vi "HardwareConfiguration.vi"() -> (3 "configured?":bool)   [LabVIEW 2018]
uses:
  InstrControl/InstrumentSetup.vi
  globals/QC_RunInformation.vi
  InstrControl/InstrControl.lvclass
panel:
  in  "Preferences Button":bool
  in  "Defaults Multimeter":bool
  in  "Multimeter":enum32{"Keithley 2000"}(tab)
  in  "Range Value\n(0.1 - 100)":dbl=100.0 format="%#.2g"
  in  "Range":u16(ring) items=["Auto", "Manual"]
  in  "Function":u16(ring)=3 items=["AC Current", "DC Current", "AC Voltage", "DC Voltage", "2W-Resistance", "4W-Resistance", "Period", "Frequency", "Temperature", "Diode", "Continuity"]
  in  "GPIB Address KE2000":string
  in  "Defaults LCR":bool
  in  "LCRs":enum32{"WayneKerr 6440B", "WayneKerr 6425"}(tab)
  in  "AC frequency [Hz]":i32=1000 format="%#.3p"
  in  "RC Configuration":u16(ring) items=["serial", "parallel"]
  in  "AC amplitude [V]":sgl=0.1
  in  "GPIB Address WK6440B":string
  in  "GPIB Address WK6425":string
  in  "AC amplitude [V] WK6425":sgl=0.1 caption="AC amplitude [V]"
  in  "RC Configuration WK6425":u16(ring) caption="RC Configuration" items=["serial", "parallel"]
  in  "AC frequency [Hz] WK6425":i32=1000 caption="AC frequency [Hz]" format="%#.3p"
  in  "VISA address":refnum<visa-resource-name>="COM24" caption="Arduino address"
  out "Programm uploaded?":string="Make sure programme is uploaded to Arduino Uno ->"
  in  "Blank Button":bool
  in  "Supplies":T1(tab)
  in  "Current Limit [µA]":sgl=100.0
  in  "GPIB Address KE2410":string
  in  "GPIB Address KE487":string
  in  "Compliance":u16(ring) items=["20µA", "2mA"]
  in  "Range:":u16(ring) items=["Autorange", "2nA", "20nA", "200nA", "2 microAmp", "20 microAmp", "200 microAmp", "2 milliAmp"]
  in  "Current Limit":u16(ring)=1 items=["OFF", "ON"]
  in  "GPIB Address KE6517":string
  in  "current compliance \nlevel [mA]":dbl=0.0001 format="%.4f"
  in  "compliance/measurement\nrange (auto:0)":u16(ring)=6 items=["auto / auto", "1 nA / 1.1 V", "10 nA / 11 V", "100 nA / 110 V", "0.001 mA / 110 V", "0.01 mA / 110 V", "0.1 mA / 110 V", "1 mA / 110 V", "10 mA / 110 V", "100 mA / 110 V"]
  in  "GPIB Address KE236":string
  in  "Defaults Supply":bool
  in  "OK Button":bool
  # "Hardware Configuration"
  # "Multimeter Configuration"
  # "Supply Configuration"
  # "Arduino Configuration"
  # "LCR Configuration"
  # "(Only for initialisation)"
  # "(Only for initialisation)"
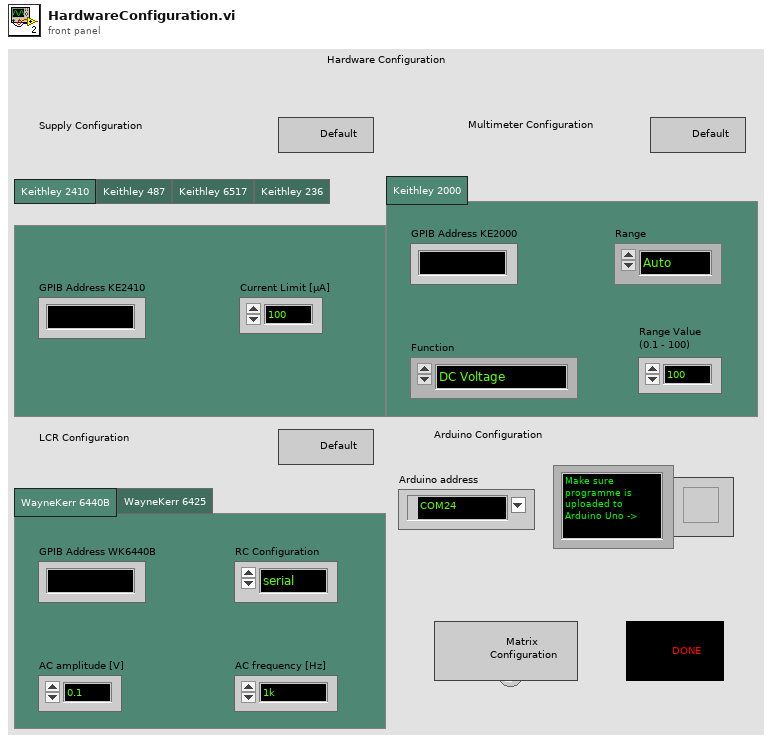
[diagram p1: front panel]
types:
  T1 = enum32{"Keithley 2410", "Keithley 487", "Keithley 6517", "Keithley 236"}
  T2 = cluster{"VISA address":refnum<visa-resource-name>, "T sensor":enum16{"SHT", "DS"}, "Arduino":refnum<class "ArduinoControl.lvclass">}
  T3 = cluster{"KE 2410":cluster{"Instrument name":string, "GPIB address":string, "Instrument type":u16}, "KE 6517":cluster{"Instrument name":string, "GPIB address":string, "Instrument type":u16}, "KE 487":cluster{"Instrument name":string, "GPIB address":string, "Instrument type":u16}, "KE 487_2":cluster{"Instrument name":string, "GPIB address":string, "Instrument type":u16}, "KE 236":cluster{"Instrument name":string, "GPIB address":string, "Instrument type":u16}, "WK 6440B":cluster{"Instrument name":string, "GPIB address":string, "Instrument type":u16}, "WK 6425":cluster{"Instrument name":string, "GPIB address":string, "Instrument type":u16}, "Pickering Matrix":cluster{"Instrument name":string, "GPIB address":string, "Instrument type":u16}, "KE 2000":cluster{"Instrument name":string, "GPIB address":string, "Instrument type":u16}, "KE 2657A":cluster{"Instrument name":string, "GPIB address":string, "Instrument type":u16}}
  T4 = cluster{"Sensor Serial No.:":string, "Wafer Serial No.:":string, "Batch:":string, "Manufacturer:":string, "Device Category:":string, "Database Serial No.:":string, "Initiated:":string, "Test":string, "Instruments used:":string, "Probeplan used:":string, "End of Run comment:":string, "User:":string}
  T5 = cluster{"RC Configuration":u16, "AC amplitude [V]":dbl, "AC frequency [Hz]":i32, "WK6440B":refnum<class "WK6440B.lvclass">}
  T6 = cluster{"RC Configuration":u16, "AC amplitude [V]":dbl, "AC frequency [Hz]":i32, "WK6425":refnum<class "WK6425.lvclass">}
  T7 = cluster{"Range":u16, "Range Value":dbl, "Function":u16, "KE2000":refnum<class "KE2000.lvclass">}
  T8 = cluster{"Current Limit":sgl, "KE2410":refnum<class "KE2410.lvclass">}
  T9 = cluster{"Compliance":u16, "Range:":u16, "KE487":refnum<class "KE487.lvclass">}
  T10 = cluster{"Current Limit":u16, "KE6517":refnum<class "KE6517.lvclass">}
  T11 = cluster{"current \ncompliance level":dbl, "compliance/\nmeasurement range (auto:0)":u16, "KE236":refnum<class "KE236.lvclass">}
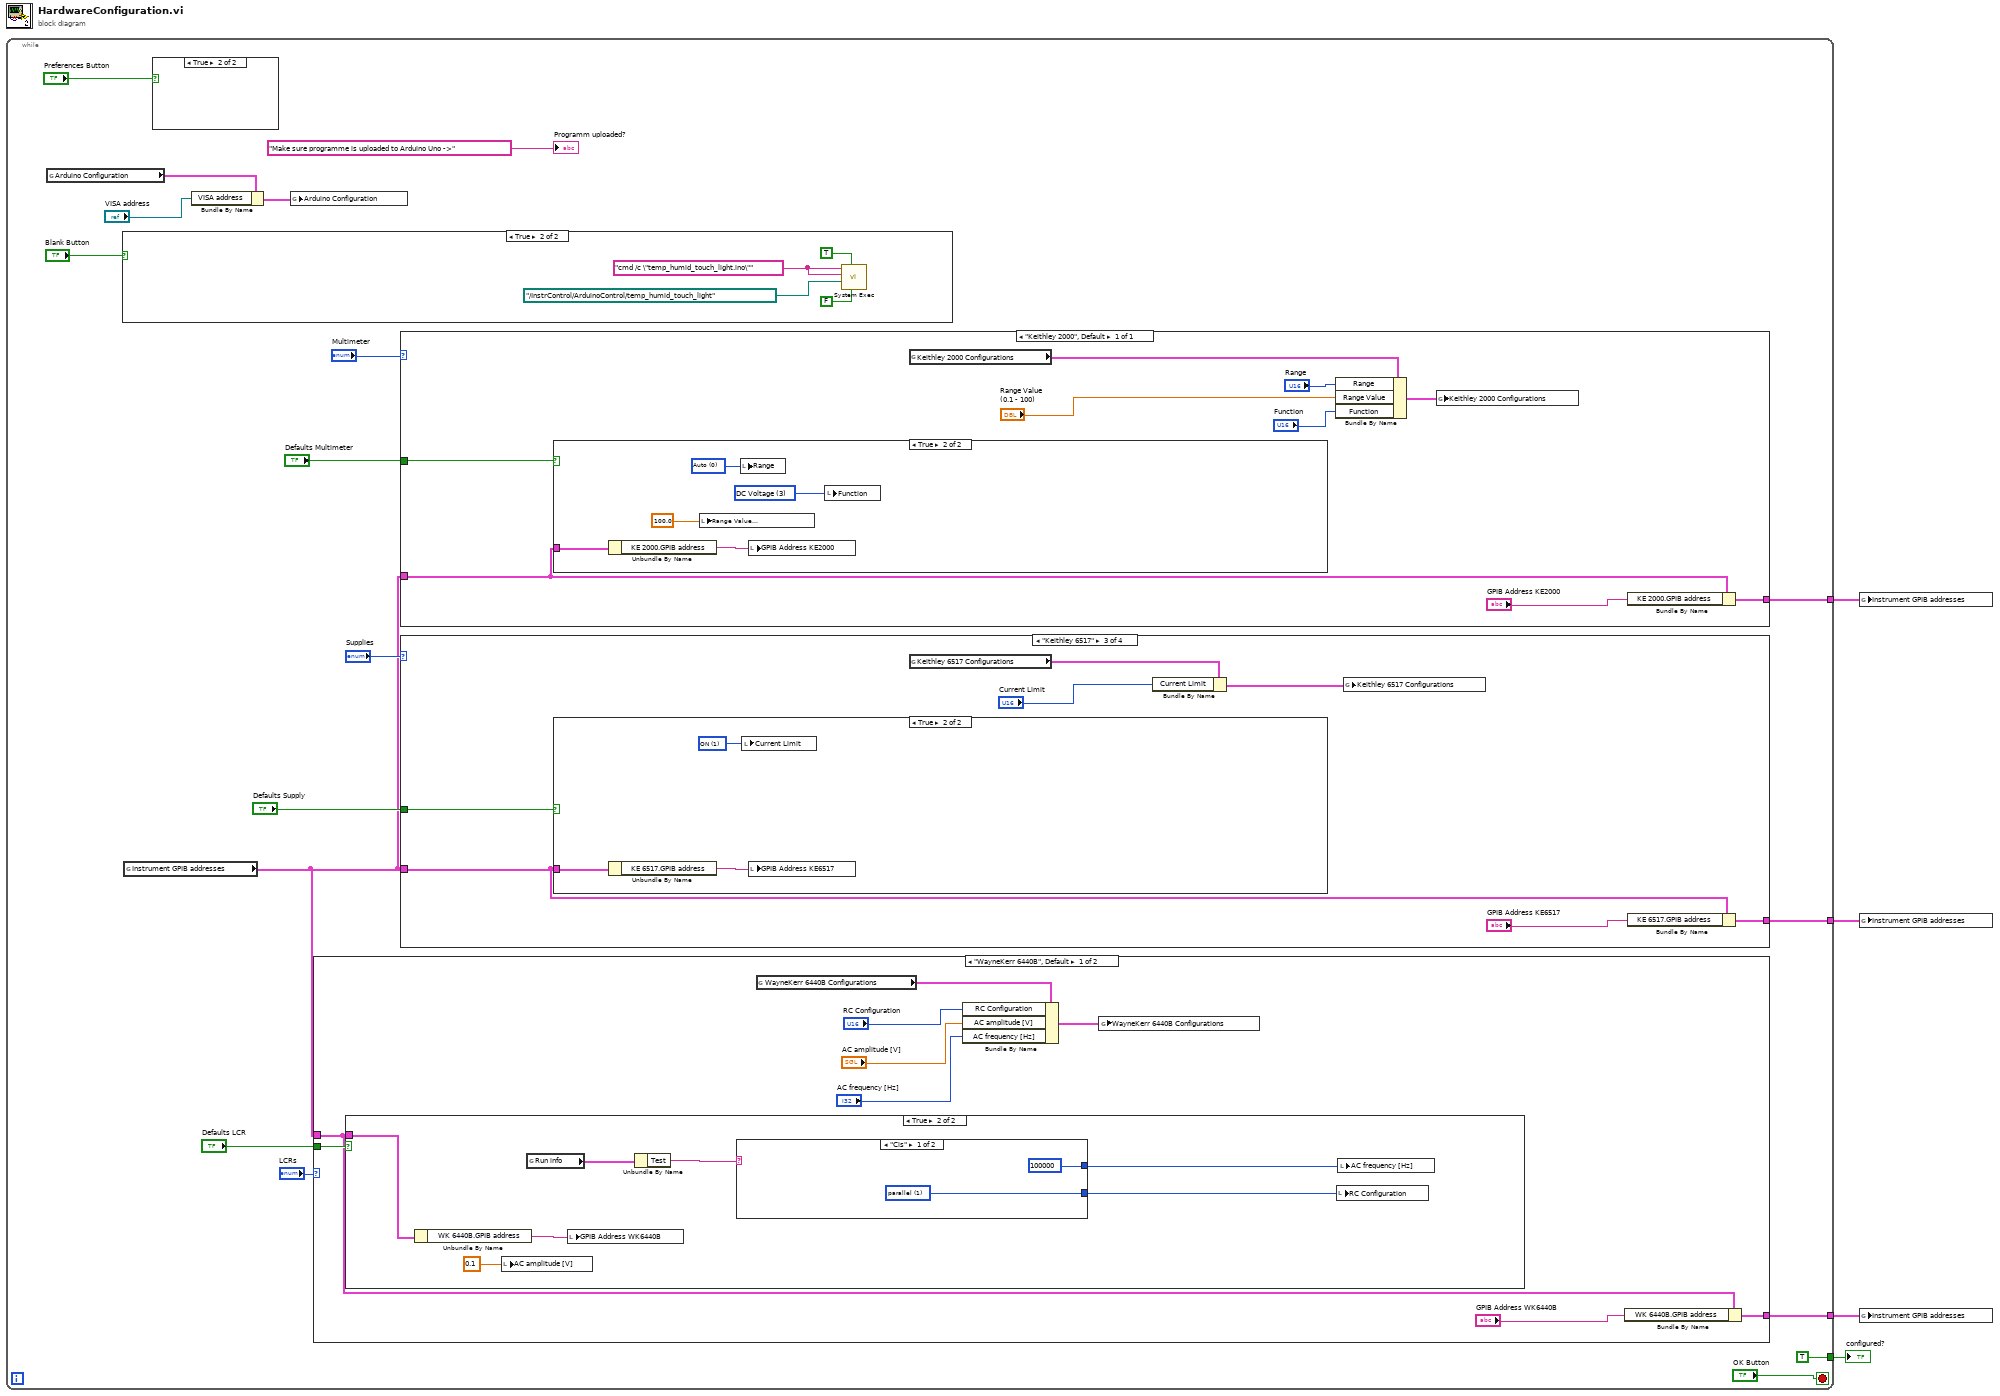
[diagram p0: block diagram]
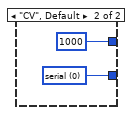
[diagram p6: hidden frame]
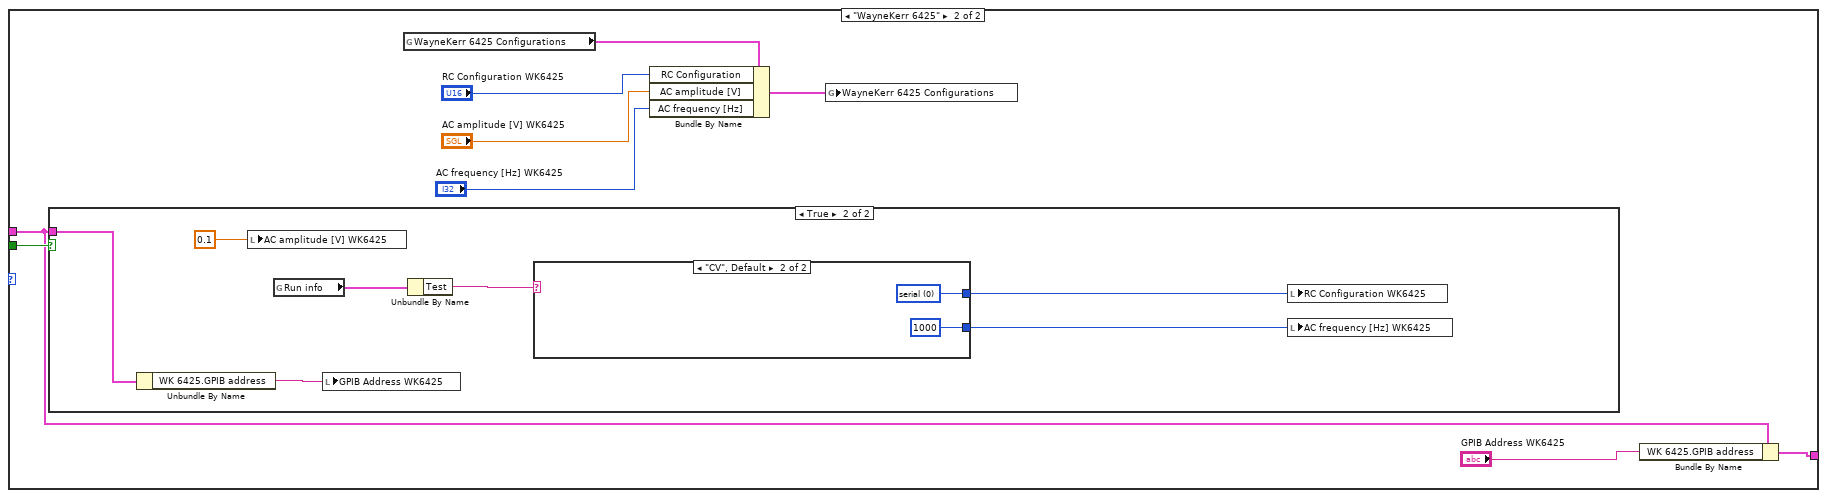
[diagram p7: hidden frame]
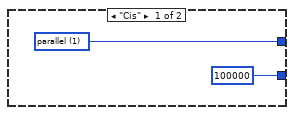
[diagram p9: hidden frame]
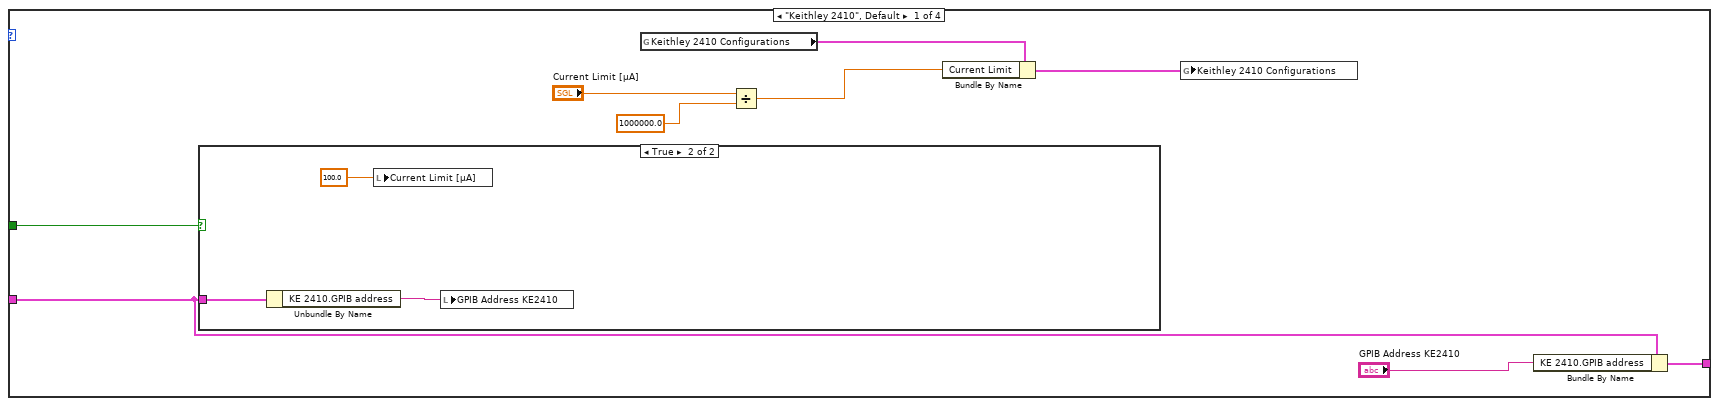
[diagram p10: hidden frame]
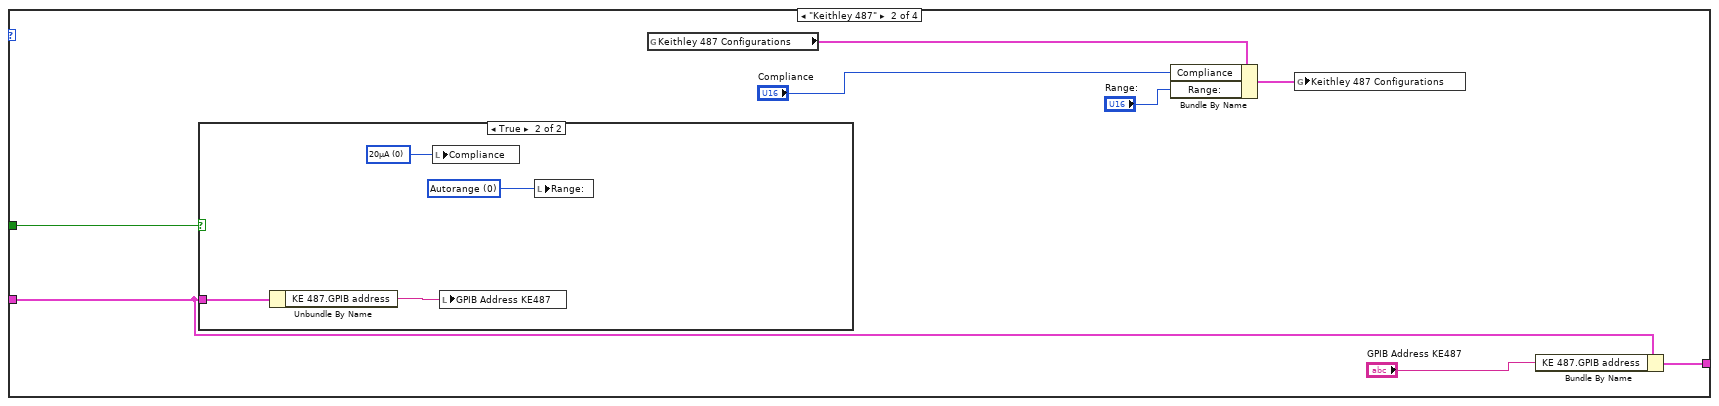
[diagram p12: hidden frame]
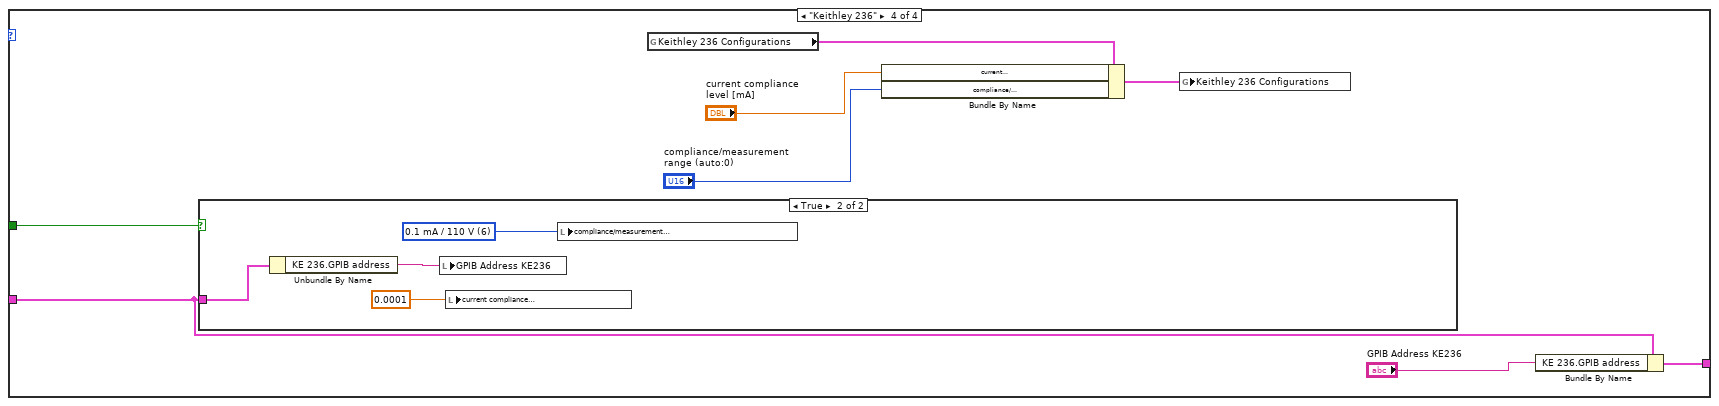
[diagram p15: hidden frame]
diagram:
  n1 = while {
    tunnel: [w9] -> w4
    tunnel: [w8] -> w3
    tunnel: [w7] -> w2
    tunnel: [TRUE] -> w1
    stop <- "OK Button" stop-if-true
    n2 = global read "InstrumentSetup.vi" "Arduino Configuration"() -> (w12:T2)
    n3 = case shown="True" "Blank Button" {
      frame False {
      }
      frame True {
        w24 = "cmd /c \"temp_humid_touch_light.ino\""
        n4 = call <vilib>:"System Exec.vi"("run minimized? (F)"=FALSE, "wait until completion? (T)"=TRUE, "working directory"=path "../InstrControl/ArduinoControl/temp_humid_touch_light", "standard input"=w24, "command line"=w24) -> ()  [unwired: 3 in, 4 out]
      }
    }
    n5 = global read "InstrumentSetup.vi" "Instrument GPIB addresses"() -> (w17:T3)
    n6 = case shown="True" "Preferences Button" {
      frame False {
      }
      frame True {
      }
    }
    n7 = Bundle By Name(cluster=w12, "VISA address"="VISA address") -> (w11:T2)
    n8 = global write "InstrumentSetup.vi" "Arduino Configuration"(w11) -> ()
    n9 = case shown="\"WayneKerr 6440B\", Default" "LCRs" {
      tunnel: "Defaults LCR" -> [w47 w67]
      tunnel: w17 -> [w46 w66]
      tunnel: [w45 w65] -> w9
      frame "WayneKerr 6440B", Default {
        n10 = case shown="True" w47 {
          tunnel: w46 -> [_ w56]
          frame False {
          }
          frame True {
            n11 = Unbundle By Name(w56) -> ("WK 6440B.GPIB address"=w50:string)
            n12 = local write "AC amplitude [V]"(0.1) -> ()
            n13 = global read "QC_RunInformation.vi" "Run info"() -> (w52:T4)
            n14 = local write "GPIB Address WK6440B"(w50) -> ()
            n15 = Unbundle By Name(w52) -> ("Test"=w51:string)
            n16 = case shown="\"Cis\"" w51 {
              tunnel: [w58 w60] -> w54
              tunnel: [100000 1000] -> w53
              frame "Cis" {
                w58 = u16 1 items=["serial", "parallel"] ("RC Configuration")
              }
              frame "CV", Default {
                w60 = u16 0 items=["serial", "parallel"] ("RC Configuration")
              }
            }
            n17 = local write "RC Configuration"(w54) -> ()
            n18 = local write "AC frequency [Hz]"(w53) -> ()
          }
        }
        n19 = global read "InstrumentSetup.vi" "WayneKerr 6440B Configurations"() -> (w49:T5)
        n20 = Bundle By Name(cluster=w49, "RC Configuration"="RC Configuration", "AC amplitude [V]"="AC amplitude [V]", "AC frequency [Hz]"="AC frequency [Hz]") -> (w48:T5)
        n21 = global write "InstrumentSetup.vi" "WayneKerr 6440B Configurations"(w48) -> ()
        n22 = Bundle By Name(cluster=w46, "WK 6440B.GPIB address"="GPIB Address WK6440B") -> (w45:T3)
      }
      frame "WayneKerr 6425" {
        n23 = case shown="True" w67 {
          tunnel: w66 -> [_ w76]
          frame False {
          }
          frame True {
            n24 = Unbundle By Name(w76) -> ("WK 6425.GPIB address"=w70:string)
            n25 = local write "AC amplitude [V] WK6425"(0.1) -> ()
            n26 = global read "QC_RunInformation.vi" "Run info"() -> (w72:T4)
            n27 = local write "GPIB Address WK6425"(w70) -> ()
            n28 = Unbundle By Name(w72) -> ("Test"=w71:string)
            n29 = case shown="\"CV\", Default" w71 {
              tunnel: [w78 w80] -> w74
              tunnel: [100000 1000] -> w73
              frame "Cis" {
                w78 = u16 1 items=["serial", "parallel"] ("RC Configuration")
              }
              frame "CV", Default {
                w80 = u16 0 items=["serial", "parallel"] ("RC Configuration")
              }
            }
            n30 = local write "RC Configuration WK6425"(w74) -> ()
            n31 = local write "AC frequency [Hz] WK6425"(w73) -> ()
          }
        }
        n32 = global read "InstrumentSetup.vi" "WayneKerr 6425 Configurations"() -> (w69:T6)
        n33 = Bundle By Name(cluster=w69, "RC Configuration"="RC Configuration WK6425", "AC amplitude [V]"="AC amplitude [V] WK6425", "AC frequency [Hz]"="AC frequency [Hz] WK6425") -> (w68:T6)
        n34 = global write "InstrumentSetup.vi" "WayneKerr 6425 Configurations"(w68) -> ()
        n35 = Bundle By Name(cluster=w66, "WK 6425.GPIB address"="GPIB Address WK6425") -> (w65:T3)
      }
    }
    n36 = case shown="\"Keithley 2000\", Default" "Multimeter" {
      tunnel: "Defaults Multimeter" -> [w35]
      tunnel: w17 -> [w32]
      tunnel: [w31] -> w7
      frame "Keithley 2000", Default {
        n37 = case shown="True" w35 {
          tunnel: w32 -> [_ w40]
          frame False {
          }
          frame True {
            w38 = u16 0 items=["Auto", "Manual"] ("Range")
            w39 = u16 3 items=["AC Current", "DC Current", "AC Voltage", "DC Voltage", "2W-Resistance", "4W-Resistance", "Period", "Frequency", "Temperature", "Diode", "Continuity"] ("Function")
            n38 = Unbundle By Name(w40) -> ("KE 2000.GPIB address"=w36:string)
            n39 = local write "Range Value\n(0.1 - 100)"(100.0 ("Range Value\n(0.1 - 100)")) -> ()
            n40 = local write "Range"(w38) -> ()
            n41 = local write "GPIB Address KE2000"(w36) -> ()
            n42 = local write "Function"(w39) -> ()
          }
        }
        n43 = global read "InstrumentSetup.vi" "Keithley 2000 Configurations"() -> (w34:T7)
        n44 = Bundle By Name(cluster=w34, "Range"="Range", "Range Value"="Range Value\n(0.1 - 100)", "Function"="Function") -> (w33:T7)
        n45 = global write "InstrumentSetup.vi" "Keithley 2000 Configurations"(w33) -> ()
        n46 = Bundle By Name(cluster=w32, "KE 2000.GPIB address"="GPIB Address KE2000") -> (w31:T3)
      }
    }
    n47 = case shown="\"Keithley 6517\"" "Supplies" {
      tunnel: "Defaults Supply" -> [w89 w100 w111 w122]
      tunnel: w17 -> [w83 w97 w108 w118]
      tunnel: [w84 w96 w107 w119] -> w8
      frame "Keithley 2410", Default {
        n48 = case shown="True" w89 {
          tunnel: w83 -> [_ w92]
          frame False {
          }
          frame True {
            n49 = Unbundle By Name(w92) -> ("KE 2410.GPIB address"=w90:string)
            n50 = local write "Current Limit [µA]"(100.0) -> ()
            n51 = local write "GPIB Address KE2410"(w90) -> ()
          }
        }
        n52 = global read "InstrumentSetup.vi" "Keithley 2410 Configurations"() -> (w88:T8)
        n53 = Divide(x="Current Limit [µA]", y=1000000.0) -> (x/y=w85:dbl)
        n54 = Bundle By Name(cluster=w88, "Current Limit"=w85) -> (w87:T8)
        n55 = global write "InstrumentSetup.vi" "Keithley 2410 Configurations"(w87) -> ()
        n56 = Bundle By Name(cluster=w83, "KE 2410.GPIB address"="GPIB Address KE2410") -> (w84:T3)
      }
      frame "Keithley 487" {
        n57 = case shown="True" w100 {
          tunnel: w97 -> [_ w104]
          frame False {
          }
          frame True {
            w102 = u16 0 items=["Autorange", "2nA", "20nA", "200nA", "2 microAmp", "20 microAmp", "200 microAmp", "2 milliAmp"] ("Range:")
            w103 = u16 0 items=["20µA", "2mA"] ("Compliance")
            n58 = Unbundle By Name(w104) -> ("KE 487.GPIB address"=w101:string)
            n59 = local write "Compliance"(w103) -> ()
            n60 = local write "GPIB Address KE487"(w101) -> ()
            n61 = local write "Range:"(w102) -> ()
          }
        }
        n62 = global read "InstrumentSetup.vi" "Keithley 487 Configurations"() -> (w99:T9)
        n63 = Bundle By Name(cluster=w99, "Compliance"="Compliance", "Range:"="Range:") -> (w98:T9)
        n64 = global write "InstrumentSetup.vi" "Keithley 487 Configurations"(w98) -> ()
        n65 = Bundle By Name(cluster=w97, "KE 487.GPIB address"="GPIB Address KE487") -> (w96:T3)
      }
      frame "Keithley 6517" {
        n66 = case shown="True" w111 {
          tunnel: w108 -> [_ w114]
          frame False {
          }
          frame True {
            w113 = u16 1 items=["OFF", "ON"] ("Current Limit")
            n67 = Unbundle By Name(w114) -> ("KE 6517.GPIB address"=w112:string)
            n68 = local write "Current Limit"(w113) -> ()
            n69 = local write "GPIB Address KE6517"(w112) -> ()
          }
        }
        n70 = global read "InstrumentSetup.vi" "Keithley 6517 Configurations"() -> (w110:T10)
        n71 = Bundle By Name(cluster=w110, "Current Limit"="Current Limit") -> (w109:T10)
        n72 = global write "InstrumentSetup.vi" "Keithley 6517 Configurations"(w109) -> ()
        n73 = Bundle By Name(cluster=w108, "KE 6517.GPIB address"="GPIB Address KE6517") -> (w107:T3)
      }
      frame "Keithley 236" {
        n74 = case shown="True" w122 {
          tunnel: w118 -> [_ w126]
          frame False {
          }
          frame True {
            w124 = u16 6 items=["auto / auto", "1 nA / 1.1 V", "10 nA / 11 V", "100 nA / 110 V", "0.001 mA / 110 V", "0.01 mA / 110 V", "0.1 mA / 110 V", "1 mA / 110 V", "10 mA / 110 V", "100 mA / 110 V"] ("compliance/\nmeasurement range (auto:0)")
            n75 = Unbundle By Name(w126) -> ("KE 236.GPIB address"=w123:string)
            n76 = local write "GPIB Address KE236"(w123) -> ()
            n77 = local write "current compliance \nlevel [mA]"(0.0001 ("current \ncompliance level")) -> ()
            n78 = local write "compliance/measurement\nrange (auto:0)"(w124) -> ()
          }
        }
        n79 = global read "InstrumentSetup.vi" "Keithley 236 Configurations"() -> (w120:T11)
        n80 = Bundle By Name(cluster=w120, "current \ncompliance level"="current compliance \nlevel [mA]", "compliance/\nmeasurement range (auto:0)"="compliance/measurement\nrange (auto:0)") -> (w121:T11)
        n81 = global write "InstrumentSetup.vi" "Keithley 236 Configurations"(w121) -> ()
        n82 = Bundle By Name(cluster=w118, "KE 236.GPIB address"="GPIB Address KE236") -> (w119:T3)
      }
    }
    "Programm uploaded?" <- "Make sure programme is uploaded to Arduino Uno ->"
  }
  "configured?" <- w1
  n83 = global write "InstrumentSetup.vi" "Instrument GPIB addresses"(w2) -> ()
  n84 = global write "InstrumentSetup.vi" "Instrument GPIB addresses"(w3) -> ()
  n85 = global write "InstrumentSetup.vi" "Instrument GPIB addresses"(w4) -> ()
